vi "editDialog.vi"(0 "reference":refnum<class "ImplicitParameterNode.lvclass">, 1 "insidePackageNode":bool, 5 "error in (no error)":errorcluster) -> (14 "reference out":refnum<class "ImplicitParameterNode.lvclass">, 15 "changeConnection":T1, 16 "cancel":bool, 19 "error out":errorcluster)   [LabVIEW 2012, in "ImplicitParameterNode.lvclass"]
doc: "Edit Dialog"
uses:
  <resource>/Framework/Providers/Open_GDS/UML/ImplicitParameterNode_class/ImplicitParameterNode.lvclass
  <resource>/Framework/Providers/Open_GDS/UML/AbstractNode_class/private/NodeConnectionStatsType.ctl
  <resource>/Framework/Providers/Open_GDS/UML/ContextHelp/ContextHelp_HelpTexts.ctl
  <resource>/Framework/Providers/Open_GDS/UML/MultiLineString_class/MultiLineString.lvclass
  <resource>/Framework/Providers/Open_GDS/UML/AbstractNode_class/AbstractNode.lvclass
panel:
  in  "Help":bool
  in  "Cancel Button":bool
  in  "OK Button":bool
  in  "Object text":string
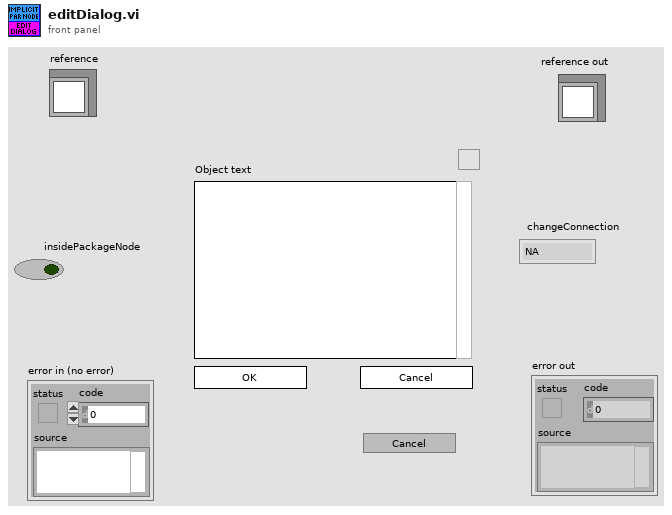
[diagram p1: front panel]
types:
  T1 = typedef "AbstractNode.lvclass/NodeConnectionStatsType.ctl" = enum16{"NA", "Connect", "DisConnect"}
  T2 = typedef "ContextHelp_HelpTexts.ctl" = enum16{"None(Hide)", "Default", "Help", "Welcome", "GettingStarted", "ClassDiagram_Help", "SequenceDiagram_Help", "UseCaseDiagram_Help", "BSelect", "BClass", "BInterface", "BPackage", "BNote", "BDependency", "BInheritance", "BInterfaceImplementation", "BAssociation", "BAggregation", "BCompAggregation", "BNoteConnector", "BObject", "BActionBar", "BCall", "BSystem", "BActor", "BUseCase", "BGeneralization", "BIncludes", "BExtends", "BUseCaseDiagramAssociation", "ClassRelationshipEdge editDialog_Bent Style", "ClassRelationshipEdge editDialog_RelationType", "ClassRelationshipEdge editDialog_Reverse association", "ClassRelationshipEdge editDialog_Start label", "ClassRelationshipEdge editDialog_Middle label", "ClassRelationshipEdge editDialog_End label", "UMLEditor reversedEngineering_Pathes", "ReversedEngineering StateReverseDialog_Help", "ReversedEngineering StateQueuedSettings_Help", "UMLEditor reversedEngineering_AddTopVIs", "UMLEditor reversedEngineering_AddClasses", "UMLEditor reversedEngineering_AddDirs", "UMLEditor reversedEngineering_Recursively", "UMLEditor reversedEngineering_Remove", "UMLEditor reversedEngineering_ClearList", "UMLEditor reversedEngineering_HideSubAss", "UMLEditor reversedEngineering_CreateTypes", "UMLEditor reversedEngineering_OnlyInheritance", "UMLEditor reversedEngineering_CreateApplication", "UMLEditor reversedEngineering_OK", "UMLEditor reversedEngineering_Cancel", "UMLEditor reversedEngineering_Help", "UMLEditor createWizardScriptFile_ScriptfilePath", "UMLEditor createWizardScriptFile_ClassPath", "UMLEditor createWizardScriptFile_Use", "UMLEditor createWizardScriptFile_PrivateDirName", "UMLEditor createWizardScriptFile_DirAppend", "UMLEditor createWizardScriptFile_Separator Character", "UMLEditor createWizardScriptFile_OK", "UMLEditor createWizardScriptFile_Cancel", "UMLEditor createWizardScriptFile_Help", "ClassNode editDialog_Class Name", "InterfaceNode editDialog_Class Name", "ClassNode editDialog_Attribute", "ClassNode editDialog_Methods", "InterfaceNode editDialog_Methods", "ClassNode editDialog_connection", "InterfaceNode editDialog_connection", "ClassNode editDialog_StereoType", "ClassNode editDialog_ShowAttrib", "ClassNode editDialog_ShowMethods", "ClassNode editDialog_ClassPath", "ClassNode editDialog_AddAttribute", "ClassNode editDialog_AddMethod", "InterfaceNode editDialog_AddMethod", "ClassNode AttributeGuide_AttributeName", "ClassNode AttributeGuide_Array?", "ClassNode AttributeGuide_Data Type", "ClassNode AttributeGuide_RefName", "ClassNode AttributeGuide_Preview", "ClassNode AttributeGuide_OK", "ClassNode AttributeGuide_Cancel", "ClassNode MethodGuide_Visibility", "ClassNode MethodGuide_Method Name", "ClassNode MethodGuide_Preview", "ClassNode MethodGuide_OK", "ClassNode MethodGuide_Cancel", "CallNode EditCallProperties_AllButtons", "ObjectNode EditObjectlProperties_AllButtons", "ActorNode EditActorProperties_AllButtons", "UseCaseRelationshipNode EditUseCaselProperties_AllButtons", "UseCaseNode EditUseCaselProperties_AllButtons", "SystemNode EditSystemProperties_AllButtons", "ReversedEngineering UpdateAttributes_AllButtons", "StateNode editDialog_AllButtons", "StateTransition editDialog_AllButtons", "ArrangeNodes Main_Picture", "ArrangeNodes Main_Zoom", "ArrangeNodes Main_Auto Zoom", "ArrangeNodes Main_shorten", "ArrangeNodes Main_Min Length", "ArrangeNodes Main_Max Length", "ArrangeNodes Main_increase", "ArrangeNodes Main_decrease", "ArrangeNodes Main_Shake", "ArrangeNodes Main", "BState", "BInitialState", "BFinalState", "BStateTransition", "StateDiagram_Help", "StateDiagram_PropertiesAllButtons", "ReversedEngineering StateReverseDialog_ClearStates", "ReversedEngineering StateReverseDialog_UseQueuedStateMachines", "ReversedEngineering StateReverseDialog_QueuedSettings", "ReversedEngineering StateReverseDialog_SearchForVIs", "ReversedEngineering StateReverseDialog_SearchCriteria", "OptionsDialog_ClassBasePath", "OptionsDialog_VIPath", "OptionsDialog_ApplicationPath", "OptionsDialog_WizDir", "OptionsDialog_IniFilePath", "OptionsDialog_DefineColors", "OptionsDialog_Help", "OptionsDialog_CreateTypes", "ClassRelationshipEdge editDialog_SplitWire"}
  T3 = typedef "ImplicitParameterNode.lvclass/ObjectAttributes.ctl" = cluster{"Base class":T4, "topHeight":dbl, "name":refnum<class "MultiLineString.lvclass">, "DEFAULT_TOP_HEIGHT":i32, "DEFAULT_WIDTH":i32, "DEFAULT_HEIGHT":i32}
  T4 = typedef "RectangularNode.lvclass/ObjectAttributes.ctl" = cluster{"Base class":T5, "bounds":T6}
  T5 = typedef "AbstractNode.lvclass/ObjectAttributes.ctl" = cluster{"parent":refnum<class "AbstractNode.lvclass">, "children":refnum<class "AbstractNode.lvclass">[], "Hidden":bool}
  T6 = typedef "Rectangle Rectangle2D.ctl" = cluster{"x":dbl, "y":dbl, "width":dbl, "height":dbl}
  T7 = typedef "ContextHelp_ShowType.ctl" = cluster{"Header":string, "Picture":picture, "Text":string}
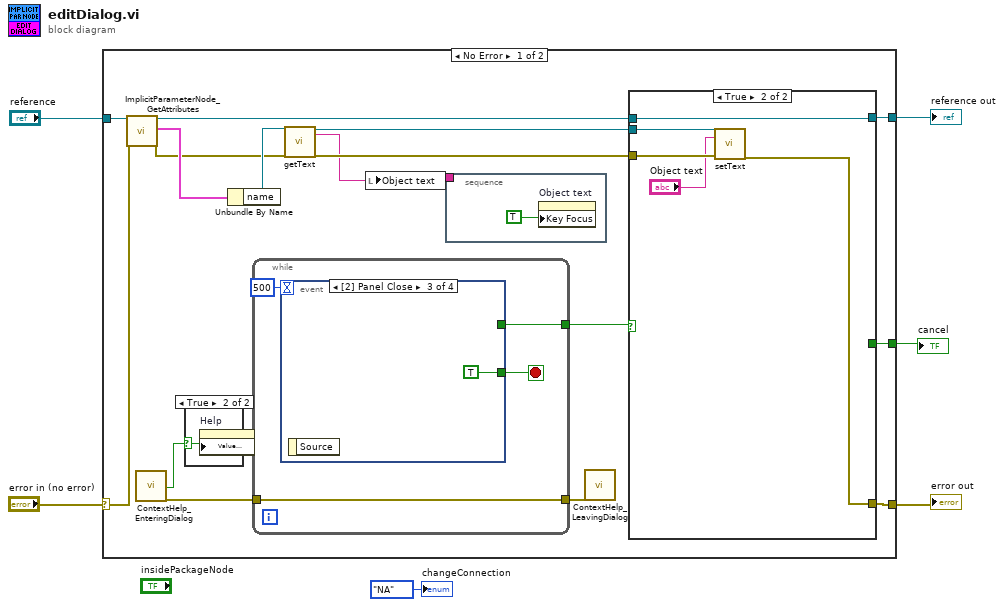
[diagram p0: block diagram]
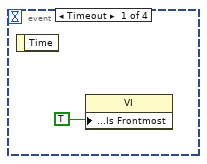
[diagram p3: hidden frame]
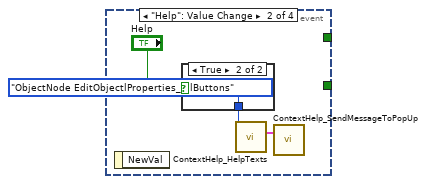
[diagram p4: hidden frame]
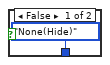
[diagram p5: hidden frame]
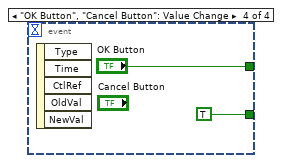
[diagram p6: hidden frame]
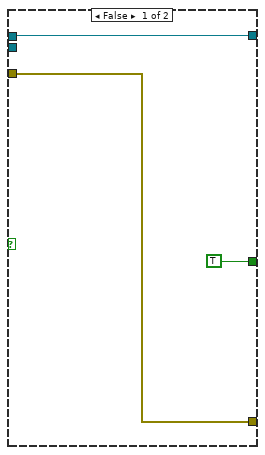
[diagram p7: hidden frame]
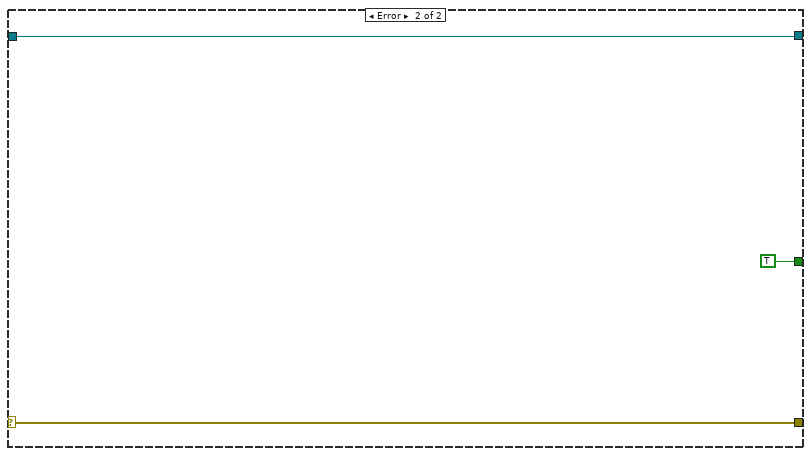
[diagram p8: hidden frame]
diagram:
  n1 = case shown="No Error" "error in (no error)" {
    selector: "error in (no error)" -> [w17 w47]
    tunnel: "reference" -> [w18 w48]
    tunnel: [w22 w47] -> w4
    tunnel: [w21 w48] -> w3
    tunnel: [w10 TRUE ("Key Focus")] -> w1
    frame No Error {
      n2 = call <resource>:"ImplicitParameterNode_GetAttributes.vi"("reference in"=w18, "error in (no error)"=w17) -> ("reference out"=w20:refnum<class "ImplicitParameterNode.lvclass">, "Attributes"=w19:T3, "error out"=w15:errorcluster)  [unwired: 15 out]
      n3 = call <resource>:"ContextHelp_EnteringDialog.vi"() -> ("HelpStatus"=w7:bool, "error out"=w8:errorcluster)  [unwired: 3 in, 15 out]
      n4 = case shown="True" w7 {
        selector: w7 -> [_ w23]
        frame False {
        }
        frame True {
          n5 = property on="Help" class="Bool (strict)"("Value (Signaling)"=w23) -> ()  [unwired: 2 in, 2 out]
        }
      }
      n6 = Unbundle By Name(w19) -> ("name"=w16:refnum<class "MultiLineString.lvclass">)
      n7 = while {
        tunnel: [w27] -> w11
        tunnel: [w25] -> w9
        tunnel: w8 -> [w25]
        stop <- w26 stop-if-true
        n8 = event shown="[2] Panel Close" {
          selector: _ -> [_ _ _ _]
          dyn-events: _ -> [_ _ _ _]
          timeout: 500 -> [_ _ _ _]
          tunnel: [_ _ _ "OK Button"] -> w27
          tunnel: [_ _ TRUE TRUE] -> w26
          event Timeout {
            n9 = event-data() -> ()  [unwired: 2 out]
            n10 = property class="VI"("Front Panel Window:Is Frontmost"=TRUE) -> ()  [unwired: 2 in, 2 out]
          }
          event "Help": Value Change {
            n11 = event-data() -> ()  [unwired: 2 out]
            n12 = case shown="True" "Help" {
              tunnel: [ContextHelp_HelpTexts."None(Hide)" ("HelpText") ContextHelp_HelpTexts."ObjectNode EditObjectlProperties_AllButtons" ("HelpText")] -> w30
              frame False {
              }
              frame True {
              }
            }
            n13 = call <resource>:"ContextHelp_HelpTexts.vi"("HelpText (enum or string)"=w30) -> ("HelpOut"=w31:T7)  [unwired: 18 out]
            n14 = call <resource>:"ContextHelp_SendMessageToPopUp.vi"("PopUpMessage"=w31) -> ()  [unwired: 2 in, 17 out]
          }
          event Panel Close {
            n15 = event-data() -> ()  [unwired: 2 out]
          }
          event "OK Button", "Cancel Button": Value Change {
            n16 = event-data() -> ()  [unwired: 6 out]
          }
        }
      }
      n17 = call-dynamic "getText.vi"("reference"=w16, "error in (no error)"=w15) -> ("reference out"=w14:refnum<class "MultiLineString.lvclass">, "text"=w12:string, "error out"=w13:errorcluster)  [unwired: 15 in]
      n18 = local write "Object text"(w12) -> ()
      n19 = stacked-sequence {
        tunnel: w12 -> [_]
        frame #0 {
          n20 = property on="Object text" class="Str"("Key Focus"=TRUE) -> ()  [unwired: 2 in, 2 out]
        }
      }
      n21 = call <resource>:"ContextHelp_LeavingDialog.vi"("error in (no error)"=w9) -> ()  [unwired: 2 in, 17 out]
      n22 = case shown="True" w11 {
        tunnel: [w38 w40] -> w22
        tunnel: [w39 w41] -> w21
        tunnel: w20 -> [w39 w41]
        tunnel: w14 -> [_ w44]
        tunnel: w13 -> [w38 w43]
        tunnel: [TRUE ("Key Focus") _] -> w10
        frame False {
        }
        frame True {
          n23 = call-dynamic "setText.vi"("reference"=w44, "text"="Object text", "error in (no error)"=w43) -> ("error out"=w40:errorcluster)  [unwired: 15 in, 1 out]
        }
      }
    }
    frame Error {
    }
  }
  "reference out" <- w3
  "error out" <- w4
  "cancel" <- w1
  "changeConnection" <- NodeConnectionStatsType."NA" ("changeConnection")
